vi "Configure List Save and Recall.vi"(8 "error in":errorcluster, 9 "File":u8=1 min=1 max=5, 10 "Type":u16(ring) items=["Save", "Recall"], 11 "VISA resource name":refnum<visa-resource-name>) -> (0 "error out":errorcluster, 3 "VISA resource name out":refnum<visa-resource-name>)   [LabVIEW 2020, in "IT-M7700.lvlib"]
doc: "This command is used to save|Recall the currently edited List file.\n<b>Type</b>\n0: Save This command is used to save the currently edited List file.\n1: Recall This command is used to invoke the saved List file.\n<b>File</b>\n1 - 5"
uses:
  <instrlib>/IT-M7700/IT-M7700.lvlib
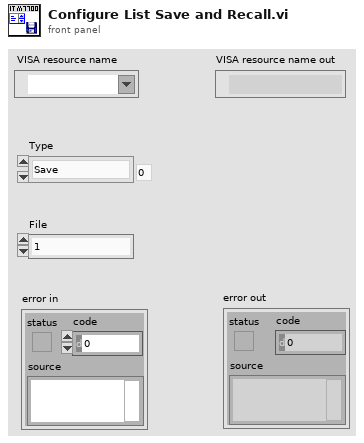
[diagram p1: front panel]
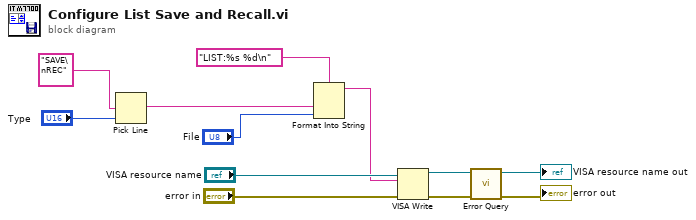
[diagram p0: block diagram]
diagram:
  n1 = Pick Line(multi-line string="SAVE\nREC", line index="Type") -> (output string=w1:string)  [unwired: 1 in]
  n2 = Format Into String(format string="LIST:%s %d\n", w1, "File") -> (resulting string=w10:string)  [unwired: 2 in, 1 out]
  n3 = VISA Write(VISA resource name="VISA resource name", write buffer=w10, error in (no error)="error in") -> (VISA resource name out=w9:refnum<visa-resource-name>, error out=w8:errorcluster)  [unwired: 1 out]
  n4 = call <instrlib>:"Error Query.vi"("error in"=w8, "VISA resource name"=w9) -> ("error out"=→"error out":errorcluster, "VISA resource name out"=→"VISA resource name out":refnum<visa-resource-name>)  [unwired: 6 in, 2 out]
